vi "SR8XX sensitivity.vi"(0 "Instrument Address":refnum<visa-resource-name>, 1 "lockin":enum16{"SRS 830", "SRS 86X", "SigRec 72XX"}(ring), 2 "set range index":u8, 3 "error in (no error)":errorcluster, 4 "read":bool) -> (5 "one step lower sensitivity":dbl format="%#_2e", 6 "one step higher sensitivity":dbl format="%#_2e", 7 "dup VISA session":refnum<visa-resource-name>, 8 "sensitivity":dbl format="%#_2e", 9 "range number":i32, 10 "error in (no error) 2":errorcluster)   [LabVIEW 2025]
doc: "This VI reads two channels of the PAR 5210 lockin. It will not work for the 5208. The output is an array of values. The input is the numeric GPIB address.\nScott Hannahs, F. Bitter National Magnet Lab, May 1993"
panel:
  out "String Returned":string
  # "set"
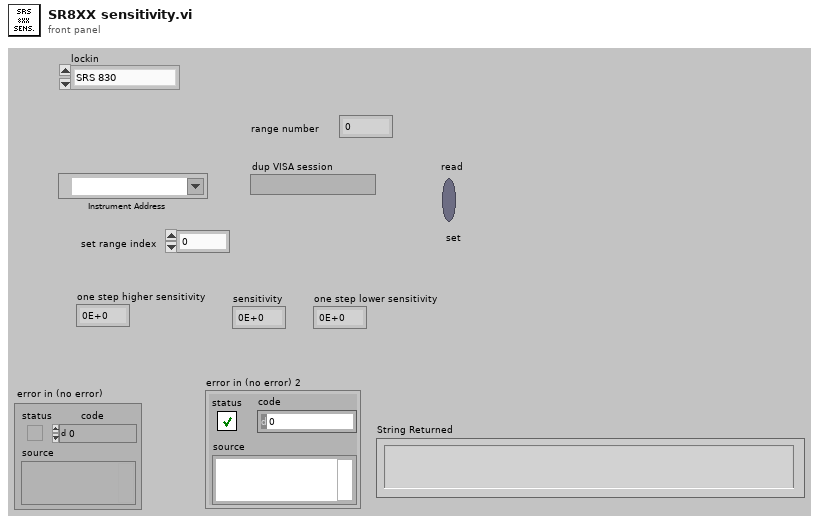
[diagram p1: front panel]
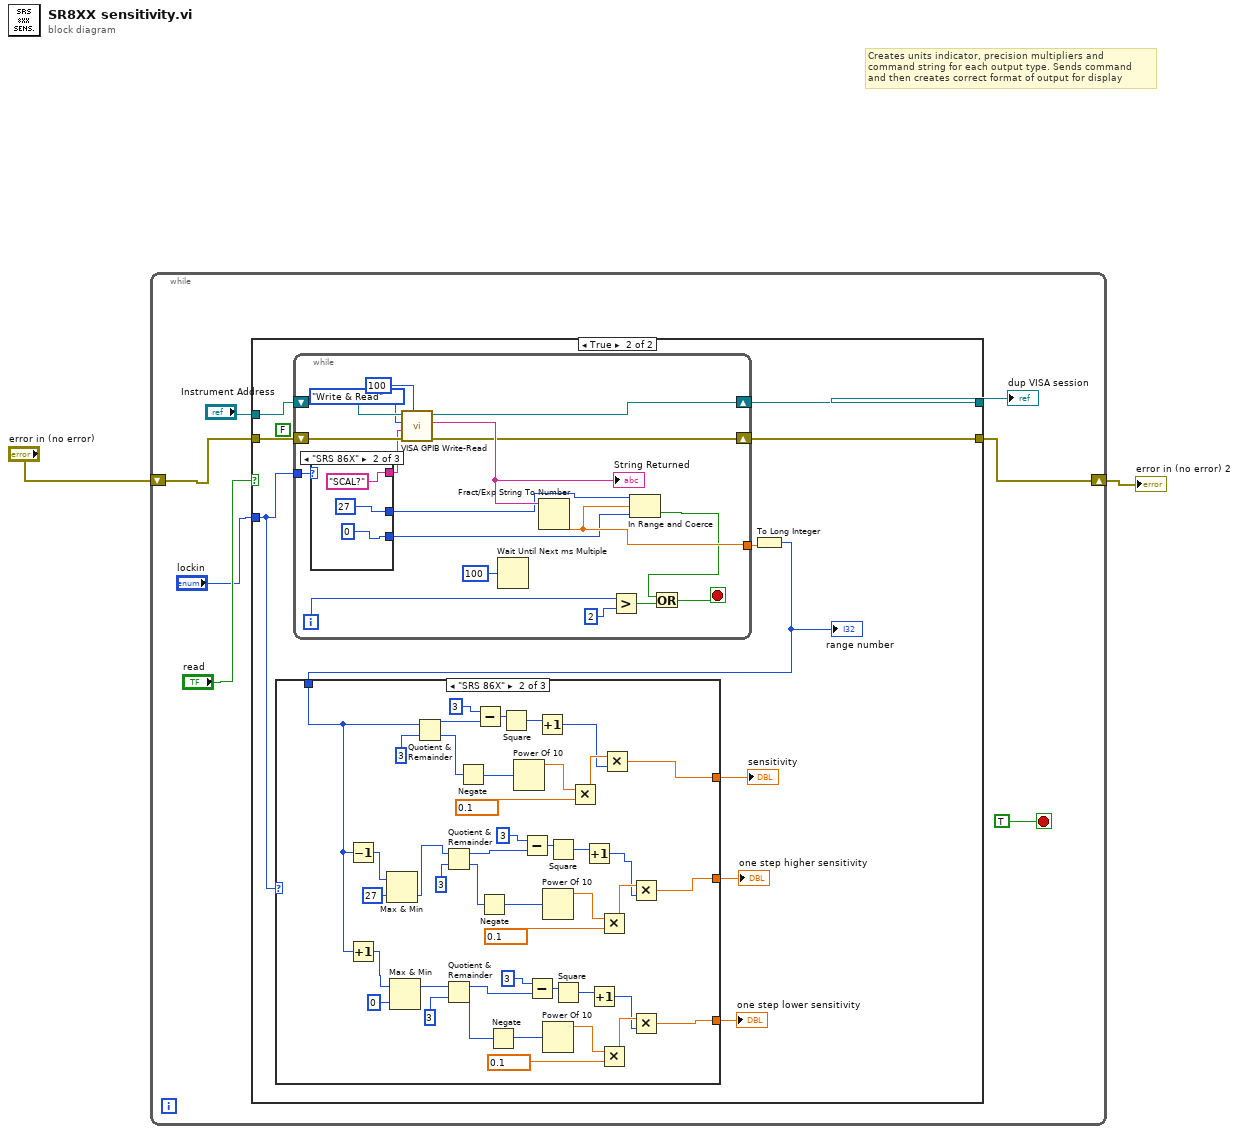
[diagram p0: block diagram]
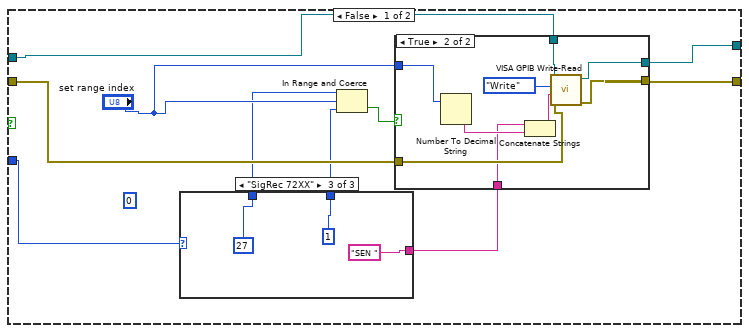
[diagram p2: hidden frame]
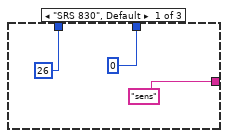
[diagram p3: hidden frame]
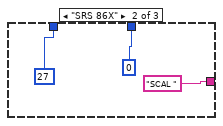
[diagram p4: hidden frame]
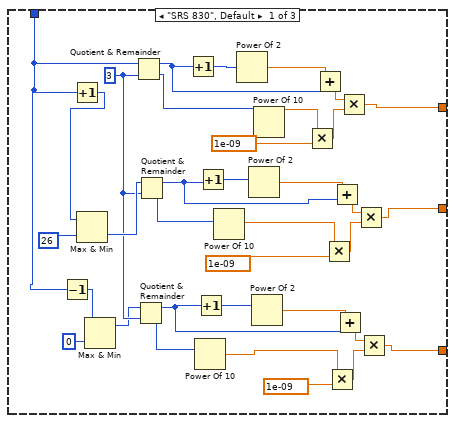
[diagram p6: hidden frame]
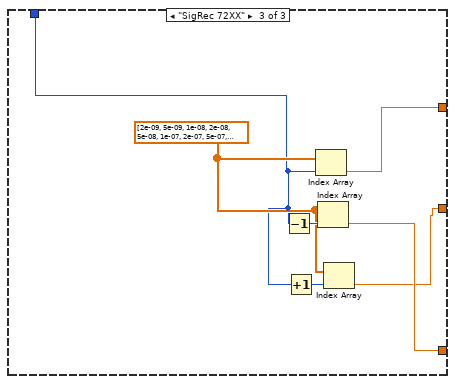
[diagram p7: hidden frame]
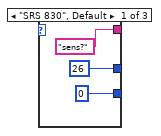
[diagram p8: hidden frame]
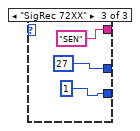
[diagram p9: hidden frame]
diagram:
  # "Creates units indicator, precision multipliers and\ncommand string for each output type. Sends command\nand then creates correct format of output for display"
  n1 = while {
    shift-right: [w6] -> w1
    shift-left: "error in (no error)" -> [w7]
    stop <- TRUE stop-if-true
    n2 = case shown="True" "read" {
      tunnel: "Instrument Address" -> [w16 w49]
      tunnel: w7 -> [w17 w48]
      tunnel: [w15 w47] -> w6
      tunnel: [w18 w46] -> w5
      tunnel: "lockin" -> [w13 w40]
      frame False {
        (unwired) u8 0 ("x")
        n3 = case shown="\"SigRec 72XX\"" w13 {
          tunnel: ["sens" ("String to Write") "SCAL " ("String to Write") "SEN " ("String to Write")] -> w12
          tunnel: [u8 0 ("lower limit") u8 0 ("lower limit") u8 1 ("lower limit")] -> w11
          tunnel: [u8 26 ("upper limit") u8 27 ("upper limit") u8 27 ("upper limit")] -> w10
          frame "SRS 830", Default {
          }
          frame "SRS 86X" {
          }
          frame "SigRec 72XX" {
          }
        }
        n4 = In Range and Coerce(upper limit=w10, x="set range index", lower limit=w11) -> (In Range?=w19:bool)  [unwired: 1 out]
        n5 = case shown="True" w19 {
          tunnel: w16 -> [w30 w38]
          tunnel: [w30 w35] -> w18
          tunnel: w17 -> [w29 w34]
          tunnel: [w29 w33] -> w15
          tunnel: "set range index" -> [_ w32]
          tunnel: w12 -> [_ w31]
          frame False {
          }
          frame True {
            n6 = Number To Decimal String(number=w32) -> (decimal integer string=w37:string)  [unwired: 1 out]
            n7 = Concatenate Strings(w31, w37) -> (w36:string)
            n8 = call "VISA GPIB Write-Read.vi"("error in (no error)"=w34, "Command"=w36, "Action"=enum16{"Write", "Read", "Write & Read"}."Write", "VISA resource name"=w38) -> ("error out"=w33:errorcluster, "dup VISA Session"=w35:refnum<visa-resource-name>)  [unwired: 4 in, 2 out]
          }
        }
      }
      frame True {
        (unwired) FALSE
        n9 = while {
          tunnel: [w139] -> w42
          shift-right: [w148] -> w46
          shift-left: w49 -> [w152]
          shift-right: [w149] -> w47
          shift-left: w48 -> [w150]
          tunnel: w40 -> [w140]
          i -> [w144]
          stop <- w141 stop-if-true
          n10 = case shown="\"SRS 86X\"" w140 {
            tunnel: ["sens?" ("String to Write") "SCAL?" ("String to Write") "SEN" ("String to Write")] -> w147
            tunnel: [u8 26 ("upper limit") u8 27 ("upper limit") u8 27 ("upper limit")] -> w136
            tunnel: [u8 0 ("lower limit") u8 0 ("lower limit") u8 1 ("lower limit")] -> w135
            frame "SRS 830", Default {
            }
            frame "SRS 86X" {
            }
            frame "SigRec 72XX" {
            }
          }
          n11 = call "VISA GPIB Write-Read.vi"("Wait (ms)"=u32 100, "error in (no error)"=w150, "Command"=w147, "Action"=enum16{"Write", "Read", "Write & Read"}."Write & Read", "VISA resource name"=w152) -> ("error out"=w149:errorcluster, "String Returned"=w151:string, "dup VISA Session"=w148:refnum<visa-resource-name>)  [unwired: 3 in, 1 out]
          "String Returned" <- w151
          n12 = Wait Until Next ms Multiple(millisecond multiple=u32 100) -> ()  [unwired: 1 out]
          n13 = Fract/Exp String To Number(string=w151) -> (number=w139:dbl)  [unwired: 3 in, 1 out]
          n14 = Greater?(x=w144, y=2) -> (0:w142:bool)
          n15 = In Range and Coerce(upper limit=w136, x=w139, lower limit=w135) -> (In Range?=w138:bool)  [unwired: 1 out]
          n16 = Or(x=w138, y=w142) -> (x .or. y?=w141:bool)
        }
        n17 = To Long Integer(number=w42) -> (32bit integer=w41:i32)
        "range number" <- w41
        n18 = case shown="\"SRS 86X\"" w40 {
          tunnel: [w76 w88 w130] -> w45
          tunnel: [w52 w87 w128] -> w44
          tunnel: [w51 w86 w129] -> w43
          tunnel: w41 -> [w50 w85 w131]
          frame "SRS 830", Default {
            w56 = u8 3 ("y")
            n19 = Decrement(x=w50) -> (x-1=w55:i32)
            n20 = Increment(x=w50) -> (x+1=w59:i32)
            n21 = Max & Min(x=w59, y=u8 26) -> (min(x,y)=w57:i32)  [unwired: 1 out]
            n22 = Max & Min(x=w55, y=u8 0) -> (max(x,y)=w53:i32)  [unwired: 1 out]
            n23 = Quotient & Remainder(x=w50, y=w56) -> (x-y*floor(x/y)=w82:i32, floor(x/y)=w77:i32)
            n24 = Quotient & Remainder(x=w53, y=w56) -> (x-y*floor(x/y)=w65:i32, floor(x/y)=w60:i32)
            n25 = Quotient & Remainder(x=w57, y=w56) -> (x-y*floor(x/y)=w73:i32, floor(x/y)=w68:i32)
            n26 = Increment(x=w82) -> (x+1=w79:i32)
            n27 = Power Of 10(x=w60) -> (10^x=w61:dbl)
            n28 = Increment(x=w65) -> (x+1=w62:i32)
            n29 = Increment(x=w73) -> (x+1=w70:i32)
            n30 = Power Of 10(x=w68) -> (10^x=w69:dbl)
            n31 = Power Of 2(x=w79) -> (2^x=w81:dbl)
            n32 = Power Of 2(x=w70) -> (2^x=w72:dbl)
            n33 = Power Of 2(x=w62) -> (2^x=w64:dbl)
            n34 = Power Of 10(x=w77) -> (10^x=w78:dbl)
            n35 = Multiply(x=w78, y=1e-09) -> (x*y=w80:dbl)
            n36 = Add(x=w81, y=w82) -> (x+y=w83:dbl)
            n37 = Multiply(x=w69, y=1e-09) -> (x*y=w71:dbl)
            n38 = Multiply(x=w61, y=1e-09) -> (x*y=w63:dbl)
            n39 = Add(x=w72, y=w73) -> (x+y=w74:dbl)
            n40 = Add(x=w64, y=w65) -> (x+y=w66:dbl)
            n41 = Multiply(x=w83, y=w80) -> (x*y=w76:dbl)
            n42 = Multiply(x=w74, y=w71) -> (x*y=w52:dbl)
            n43 = Multiply(x=w66, y=w63) -> (x*y=w51:dbl)
          }
          frame "SRS 86X" {
            n44 = Decrement(x=w85) -> (x-1=w127:i32)
            n45 = Increment(x=w85) -> (x+1=w125:i32)
            n46 = Max & Min(x=w127, y=u8 27) -> (min(x,y)=w110:i32)  [unwired: 1 out]
            n47 = Max & Min(x=w125, y=u8 0) -> (max(x,y)=w111:i32)  [unwired: 1 out]
            n48 = Quotient & Remainder(x=w85, y=u8 3) -> (x-y*floor(x/y)=w101:i32, floor(x/y)=w109:i32)
            n49 = Quotient & Remainder(x=w110, y=u8 3) -> (x-y*floor(x/y)=w95:i32, floor(x/y)=w107:i32)
            n50 = Quotient & Remainder(x=w111, y=u8 3) -> (x-y*floor(x/y)=w90:i32, floor(x/y)=w106:i32)
            n51 = Negate(x=w109) -> (-x=w108:i32)
            n52 = Subtract(x=3, y=w101) -> (x-y=w99:i32)
            n53 = Negate(x=w107) -> (-x=w104:i32)
            n54 = Negate(x=w106) -> (-x=w105:i32)
            n55 = Square(x=w99) -> (x^2=w102:i32)
            n56 = Power Of 10(x=w108) -> (10^x=w122:dbl)
            n57 = Subtract(x=3, y=w95) -> (x-y=w96:i32)
            n58 = Subtract(x=3, y=w90) -> (x-y=w91:i32)
            n59 = Increment(x=w102) -> (x+1=w103:i32)
            n60 = Power Of 10(x=w104) -> (10^x=w118:dbl)
            n61 = Power Of 10(x=w105) -> (10^x=w114:dbl)
            n62 = Square(x=w96) -> (x^2=w98:i32)
            n63 = Square(x=w91) -> (x^2=w93:i32)
            n64 = Multiply(x=w122, y=0.1) -> (x*y=w121:dbl)
            n65 = Increment(x=w98) -> (x+1=w94:i32)
            n66 = Increment(x=w93) -> (x+1=w89:i32)
            n67 = Multiply(x=w118, y=0.1) -> (x*y=w117:dbl)
            n68 = Multiply(x=w114, y=0.1) -> (x*y=w113:dbl)
            n69 = Multiply(x=w121, y=w103) -> (x*y=w88:dbl)
            n70 = Multiply(x=w117, y=w94) -> (x*y=w87:dbl)
            n71 = Multiply(x=w113, y=w89) -> (x*y=w86:dbl)
          }
          frame "SigRec 72XX" {
            w132 = dbl[] [2e-09, 5e-09, 1e-08, 2e-08, 5e-08, 1e-07, 2e-07, 5e-07, 1e-06, 2e-06, 5e-06, 1e-05, 2e-05, 5e-05, 0.0001, 0.0002, 0.0005, 0.001, 0.002, 0.005, 0.01, 0.02, 0.05, 0.1, 0.2, 0.5, 1.0] ("Array")
            n72 = Decrement(x=w131) -> (x-1=w134:i32)
            n73 = Increment(x=w131) -> (x+1=w133:i32)
            n74 = Index Array(array=w132, index=w131) -> (element=w130:dbl)
            n75 = Index Array(array=w132, index=w134) -> (element=w129:dbl)
            n76 = Index Array(array=w132, index=w133) -> (element=w128:dbl)
          }
        }
        "sensitivity" <- w45
        "one step lower sensitivity" <- w43
        "one step higher sensitivity" <- w44
      }
    }
    "dup VISA session" <- w5
  }
  "error in (no error) 2" <- w1
